vi "PixelLIDAR_Open.vi"() -> (2 "error out":errorcluster, 3 "initialized LIDAR\narray":i32[](array[numeric]), 4 "MDF Image":T1(plugin-control), 5 "MissionMap":path)   [LabVIEW 2010]
doc: "This SubVI sets up the memory space for the Lidars's MDF file and reads the MDF file into it. It is designed to run before Pixel_LIDAR_Run.VI."
panel:
  out "Y Resolution":i32
  out "X Resolution":i32
  # "This SubVI is used with PixelLIDAR_Run.VI and reads thw Mission Map file and sets up memory to accomidate it"
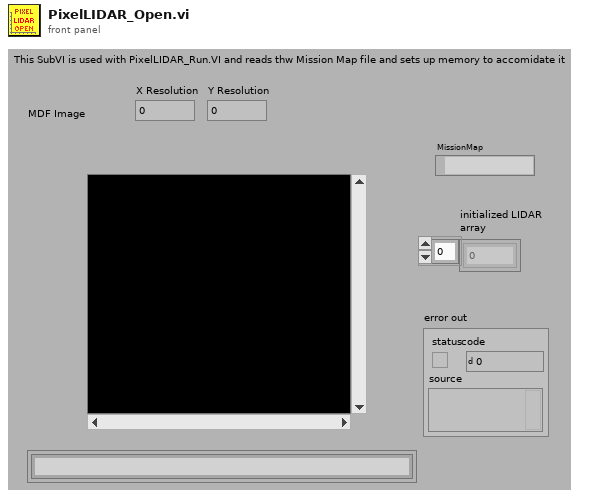
[diagram p1: front panel]
types:
  T1 = typedef "IMAQ Image.ctl" = refnum<image>
  T2 = typedef "Image Type" = u32
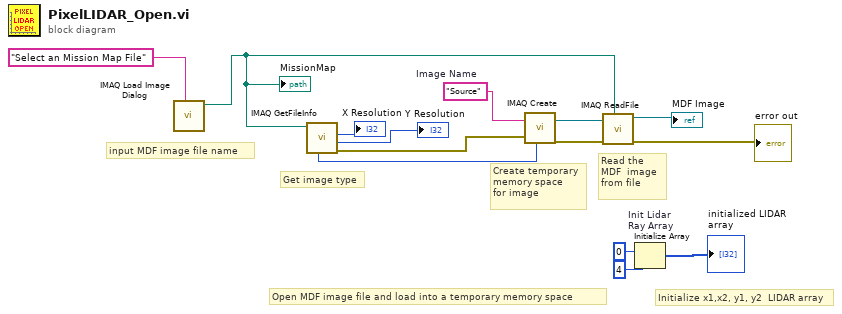
[diagram p0: block diagram]
diagram:
  w11 = "Source"  # Image Name
  # "Initialize x1,x2, y1, y2  LIDAR array"
  # "input MDF image file name"
  # "Get image type"
  # "Read the\nMDF  image\nfrom file"
  # "Create temporary\nmemory space \nfor image"
  # "Open MDF image file and load into a temporary memory space"
  n1 = call "IMAQ Load Image Dialog"("Prompt"="Select an Mission Map File" ("prompt")) -> ("Path"=w1:path)  [unwired: 6 in, 4 out]
  "MissionMap" <- w1
  n2 = call "IMAQ GetFileInfo"("File Path"=w1) -> ("error out"=w12:errorcluster, "Y Resolution"=→"Y Resolution":i32, "X Resolution"=→"X Resolution":i32, "Image Type"=w8:T2)  [unwired: 1 in, 6 out]
  n3 = call "IMAQ Create"("Image Name"=w11, "Image Type"=w8, "error in (no error)"=w12) -> ("New Image"=w13:T1, "error out"=w14:errorcluster)  [unwired: 1 in, 1 out]
  n4 = call "IMAQ ReadFile"("File Path"=w1, "error in (no error)"=w14, "Image"=w13) -> ("error out"=→"error out":errorcluster, "Image Out"=→"MDF Image":T1)  [unwired: 2 in, 5 out]
  n5 = Initialize Array "Init Lidar\nRay Array"(0 ("element"), 4 ("dimension size")) -> (→"initialized LIDAR\narray":i32[])
